vi "get period.vi"(8 "error in":errorcluster, 11 "timing source in":refnum<class "DAQmx Single Point HW Timed.lvclass">) -> (0 "error out":errorcluster, 2 "period (ns)":i64, 3 "timing source out":refnum<class "DAQmx Single Point HW Timed.lvclass">)   [LabVIEW 2014, in "DAQmx Single Point HW Timed.lvclass"]
doc: "Returns the rate of the clock used by the selected timing source. This rate is the period measured in nanoseconds.\n\nIf the timing source has an unknown period, return -1."
uses:
  DAQmx Single Point HW Timed.lvclass
  <vilib>/NI/Module Timing Source/timing source/TBM timing source.lvclass
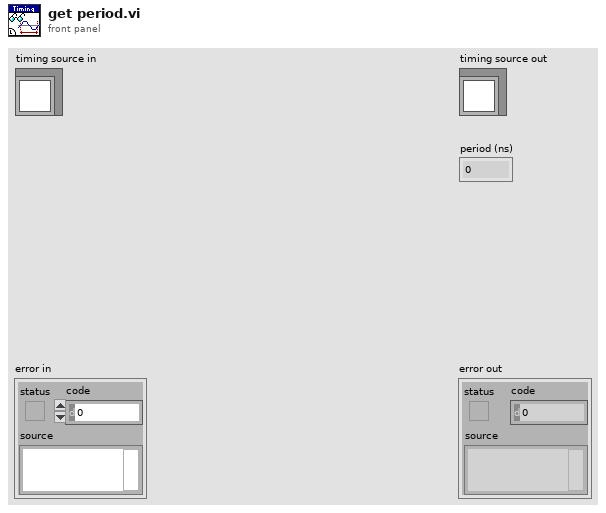
[diagram p1: front panel]
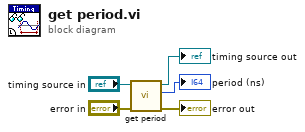
[diagram p0: block diagram]
diagram:
  n1 = call-parent "get period.vi"("error in"="error in", "timing source in"="timing source in") -> ("error out"=→"error out":errorcluster, "period (ns)"=→"period (ns)":i64, "timing source out"=→"timing source out":refnum<class "DAQmx Single Point HW Timed.lvclass">)  [unwired: 7 in]
